vi "FTW-Endpoint-Multipart-Send.vi"(0 "FTW Endpoint":refnum<class "FTW-Endpoint.lvclass">, 5 "Message":T1, 7 "Timeout":i32 format="%dmsec", 11 "error in":errorcluster) -> (4 "FTW Endpoint out":refnum<class "FTW-Endpoint.lvclass">, 6 "Timed out?":bool, 15 "error out":errorcluster)   [LabVIEW 2013, in "FTW-Endpoint.lvclass"]
uses:
  FTW-Endpoint.lvclass
  Payload/FTW-MessagePayload.ctl
  FTW-Endpoint.lvclass/FTW-Endpoint.ctl
panel:
  # "Inputs"
  # "Outputs"
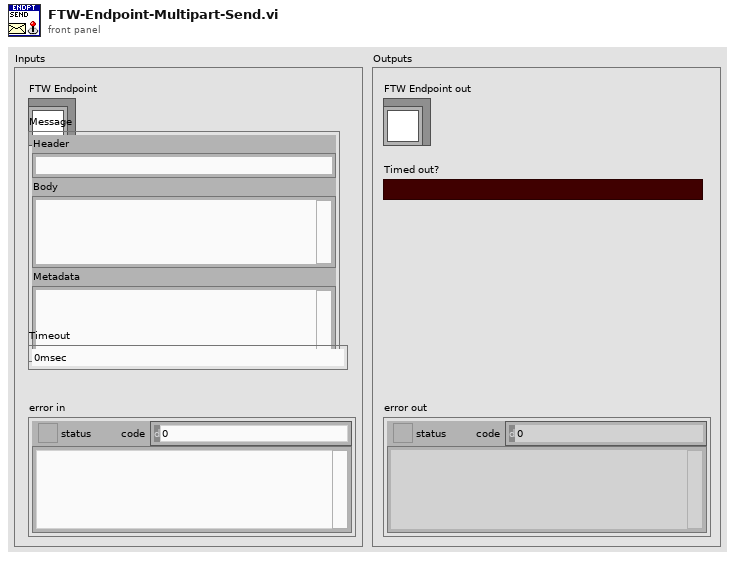
[diagram p1: front panel]
types:
  T1 = typedef "FTW-MessagePayload.ctl" = cluster{"Header":string, "Body":string, "Metadata":string}
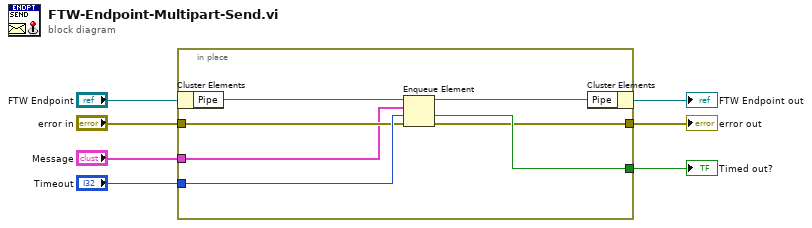
[diagram p0: block diagram]
diagram:
  n1 = in-place {
    in-place-border: [w14] -> w2
    in-place-border: "Timeout" -> [w13]
    in-place-border: "error in" -> [w12]
    in-place-border: [w11] -> w7
    in-place-border: "Message" -> [w10]
    n2 = in-place-cluster #1("FTW Endpoint") -> ("Pipe"=w9:refnum<queue>)
    n3 = Enqueue Element(queue=w9, element=w10, timeout in ms (-1)=w13, error in (no error)=w12) -> (queue out=w8:refnum<queue>, timed out?=w14:bool, error out=w11:errorcluster)
    n4 = in-place-cluster #1("Pipe"=w8) -> (→"FTW Endpoint out":refnum<class "FTW-Endpoint.lvclass">)
  }
  "error out" <- w7
  "Timed out?" <- w2
